vi "Find Network Systems.vi"(8 "Error IN":errorcluster caption="error in (no error)") -> (0 "Error OUT":errorcluster caption="error in (no error)", 3 "Serial Number":u32)   [LabVIEW 2013]
uses:
  Type Defs/TCP Data Stream Mode (PC).ctl
  <vilib>/nisyscfg/Find Hardware.vi
  <vilib>/nisyscfg/Close (System).vi
  <vilib>/nisyscfg/nisyscfg.lvlib
  <resource>/objmgr/nisysapi.rc
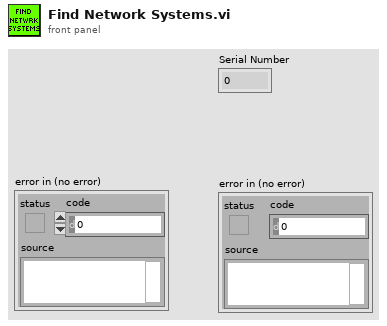
[diagram p1: front panel]
types:
  T1 = typedef "TCP Data Stream Mode (PC).ctl" = enum16{"Init", "Read Data", "Close"}
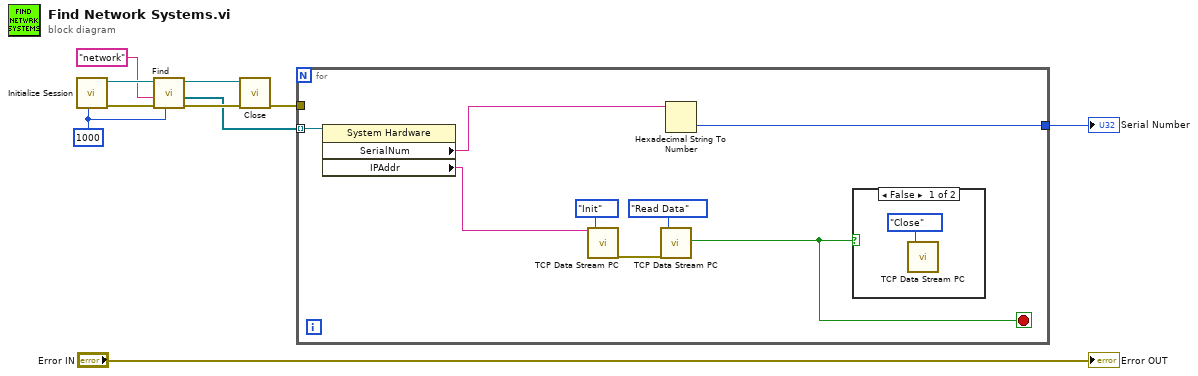
[diagram p0: block diagram]
diagram:
  w5 = u32 1000 ("connect timeout in ms (4s)")
  n1 = call <vilib>:"Initialize Session.vi"("connect timeout in ms (4s)"=w5) -> ("error out"=w6:errorcluster, "session out"=w10:refnum<k21>)  [unwired: 9 in]
  n2 = call-poly <vilib>:"Find.vi"("remote timeout in ms (5m)"=w5, "error in (no error)"=w6, "experts"="network", "session in"=w10) -> ("error out"=w8:errorcluster, "resources out"=w7:refnum<k20>[], "session out"=w9:refnum<k21>)  [unwired: 4 in, 1 out]
  n3 = call-poly <vilib>:"Close.vi"("error in (no error)"=w8, "session in"=w9) -> ("error out"=w4:errorcluster)  [unwired: 9 in]
  n4 = for {
    tunnel: w7 -> [w18] mode=indexing
    tunnel: w4 -> [_]
    tunnel: [w16] -> w2
    stop <- w11 stop-if-true
    n5 = property class="System Hardware"(reference=w18) -> ("SerialNum"=w17:string, "IPAddr"=w12:string)  [unwired: 1 in, 2 out]
    n6 = call "TCP Data Stream PC.vi"("RT IP Address"=w12, "Mode"=TCP_Data_Stream_Mode_(PC)."Init") -> ("Error OUT"=w13:errorcluster)  [unwired: 14 in, 3 out]
    n7 = call "TCP Data Stream PC.vi"("Error IN"=w13, "Mode"=TCP_Data_Stream_Mode_(PC)."Read Data") -> ("Connected?"=w11:bool)  [unwired: 14 in, 3 out]
    n8 = Hexadecimal String To Number(string=w17) -> (number=w16:u32)  [unwired: 2 in, 1 out]
    n9 = case shown="False" w11 {
      frame False {
        n10 = call "TCP Data Stream PC.vi"("Mode"=TCP_Data_Stream_Mode_(PC)."Close") -> ()  [unwired: 15 in, 4 out]
      }
      frame True {
      }
    }
  }
  "Serial Number" <- w2
  "Error OUT" <- "Error IN"
